vi "Cholesky Factorization Rank-1 Update.vi"   [LabVIEW 2020, in "NI_AAL_LinAlg.lvlib"]
doc: "Performs Cholesky factorization on the rank-1 updated Cholesky matrix. The VI performs Cholesky factorization directly on the known factored matrix instead of the updated matrix."
uses:
  <vilib>/Analysis/NI_AAL_LinAlg.lvlib
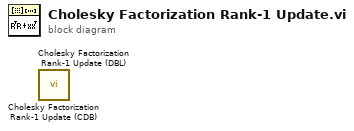
[diagram p0: block diagram]
diagram:
  n1 = call <vilib>:"Cholesky Factorization Rank-1 Update (CDB).vi"() -> ()  [unwired: 10 in, 2 out]
  n2 = call <vilib>:"Cholesky Factorization Rank-1 Update (DBL).vi"() -> ()  [unwired: 10 in, 2 out]
